vi "生成校准信息.vi"(5 "量程选择":enum16{"低量程", "高量程"}(ring), 7 "公式系数":dbl[](array[numeric]), 8 "启用":bool[](array[boolean]), 9 "校准时间":string[](array[string]), 10 "信号值":dbl[](array[numeric]), 11 "校准浓度":dbl[](array[numeric])) -> ()   [LabVIEW 2016, in "斯坦道CODMn.lvlib"]
panel:
  out "data":T1
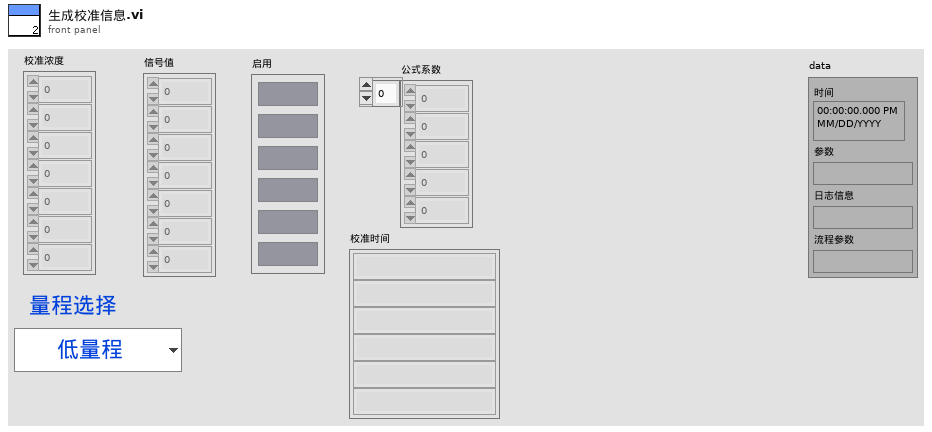
[diagram p1: front panel]
types:
  T1 = typedef "操作日志字段定义.ctl" = cluster{"时间":timestamp, "参数":string, "日志信息":string, "流程参数":string}
  T2 = cluster{"低标液1浓度":dbl, "低标液1信号值":dbl, "低标液1启用":u16, "低标液2浓度":dbl, "低标液2信号值":dbl, "低标液2启用":u16, "低标液3浓度":dbl, "低标液3信号值":dbl, "低标液3启用":u16, "低标液4浓度":dbl, "低标液4信号值":dbl, "低标液4启用":u16, "低标液5浓度":dbl, "低标液5信号值":dbl, "低标液5启用":u16, "高标液1浓度":dbl, "高标液1信号值":dbl, "高标液1启用":u16, "高标液2浓度":dbl, "高标液2信号值":dbl, "高标液2启用":u16, "高标液3浓度":dbl, "高标液3信号值":dbl, "高标液3启用":u16, "高标液4浓度":dbl, "高标液4信号值":dbl, "高标液4启用":u16, "高标液5浓度":dbl, "高标液5信号值":dbl, "高标液5启用":u16}
  T3 = cluster{"[0]":string, "[1]":string, "[2]":string}
  T4 = cluster{"时间标识":timestamp, "参数":string, "日志信息":string, "流程参数":string}
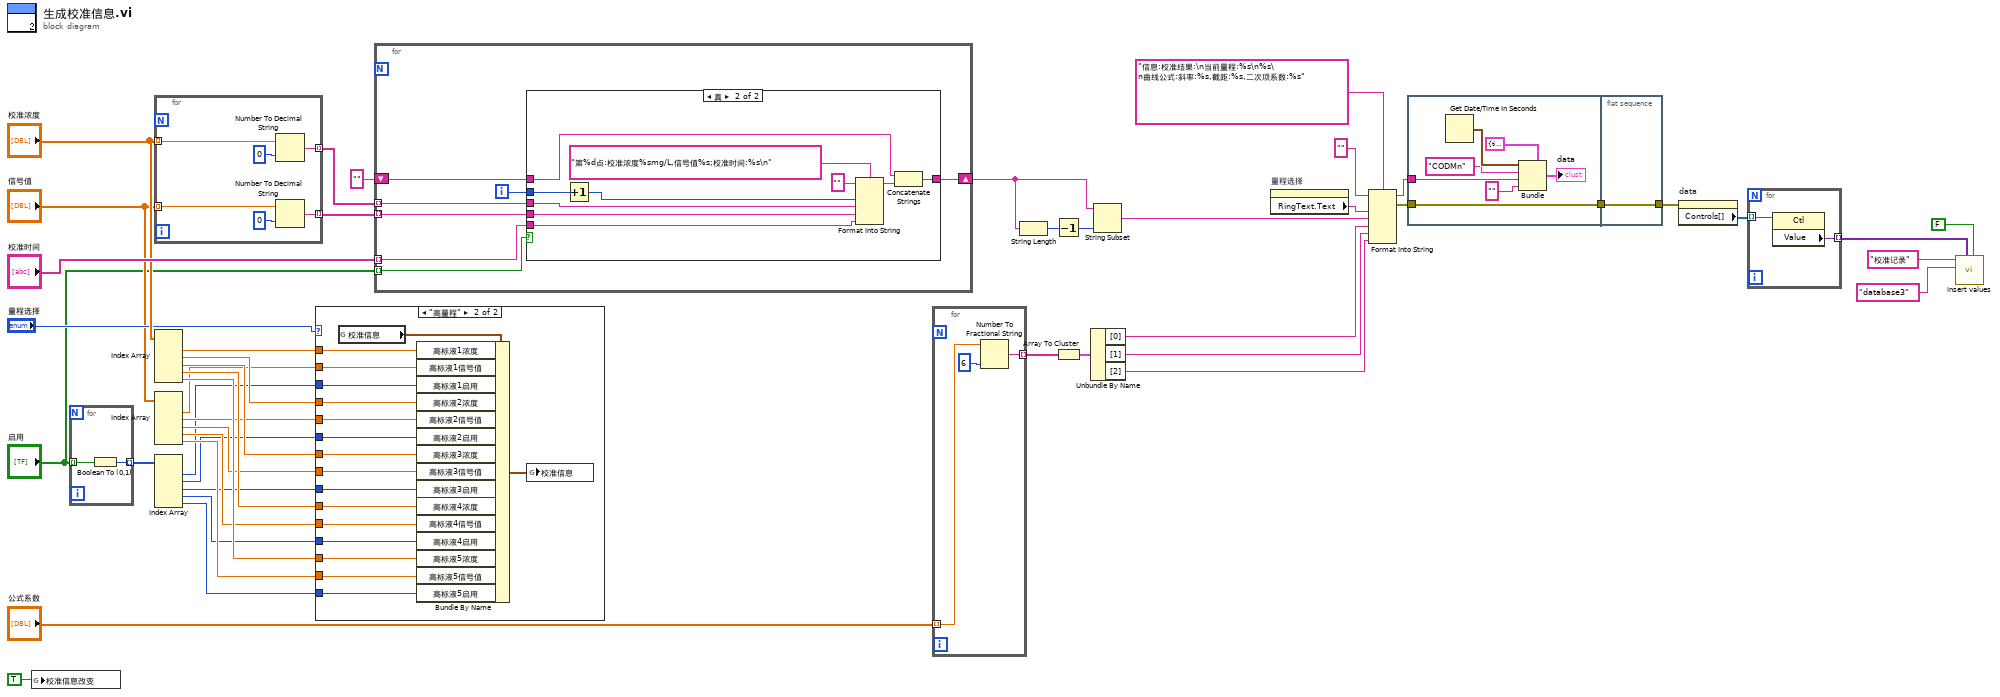
[diagram p0: block diagram]
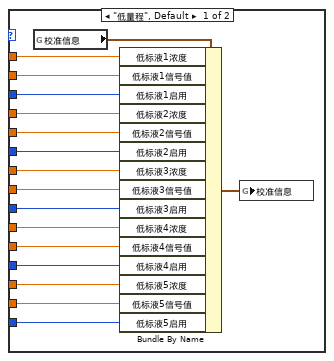
[diagram p2: hidden frame]
diagram:
  n1 = global write "CODMn断电保存全局变量.vi" "校准信息改变"(TRUE ("校准信息改变")) -> ()
  n2 = for {
    tunnel: "启用" -> [w49] mode=indexing
    tunnel: [w48] -> w6 mode=indexing
    n3 = Boolean To (0,1)(Boolean=w49) -> (0, 1=w48:i16)
  }
  n4 = for {
    tunnel: "校准浓度" -> [w55] mode=indexing
    tunnel: "信号值" -> [w52] mode=indexing
    tunnel: [w51] -> w25 mode=indexing
    tunnel: [w50] -> w24 mode=indexing
    n5 = Number To Decimal String(number=w55, width (-)=i16 0 ("宽度(-)")) -> (decimal integer string=w51:string)
    n6 = Number To Decimal String(number=w52, width (-)=i16 0 ("宽度(-)")) -> (decimal integer string=w50:string)
  }
  n7 = Index Array(array="校准浓度") -> (element #1=w18:dbl, element #2=w17:dbl, element #3=w16:dbl, element #4=w15:dbl, element #5=w14:dbl)  [unwired: 5 in]
  n8 = Index Array(array="信号值") -> (element #1=w12:dbl, element #2=w11:dbl, element #3=w10:dbl, element #4=w9:dbl, element #5=w8:dbl)  [unwired: 5 in]
  n9 = Index Array(array=w6) -> (element #1=w5:i16, element #2=w4:i16, element #3=w3:i16, element #4=w2:i16, element #5=w1:i16)  [unwired: 5 in]
  n10 = case shown="\"高量程\"" "量程选择" {
    tunnel: w18 -> [w70 w87]
    tunnel: w17 -> [w69 w86]
    tunnel: w16 -> [w68 w85]
    tunnel: w15 -> [w67 w84]
    tunnel: w14 -> [w66 w83]
    tunnel: w12 -> [w65 w78]
    tunnel: w11 -> [w64 w79]
    tunnel: w10 -> [w63 w80]
    tunnel: w9 -> [w62 w81]
    tunnel: w8 -> [w61 w82]
    tunnel: w5 -> [w56 w77]
    tunnel: w4 -> [w57 w76]
    tunnel: w3 -> [w58 w75]
    tunnel: w2 -> [w59 w74]
    tunnel: w1 -> [w60 w73]
    frame "低量程", Default {
      n11 = global read "CODMn断电保存全局变量.vi" "校准信息"() -> (w71:T2)
      n12 = Bundle By Name(cluster=w71, "低标液1浓度"=w70, "低标液1信号值"=w65, "低标液1启用"=w56, "低标液2浓度"=w69, "低标液2信号值"=w64, "低标液2启用"=w57, "低标液3浓度"=w68, "低标液3信号值"=w63, "低标液3启用"=w58, "低标液4浓度"=w67, "低标液4信号值"=w62, "低标液4启用"=w59, "低标液5浓度"=w66, "低标液5信号值"=w61, "低标液5启用"=w60) -> (w72:T2)
      n13 = global write "CODMn断电保存全局变量.vi" "校准信息"(w72) -> ()
    }
    frame "高量程" {
      n14 = global read "CODMn断电保存全局变量.vi" "校准信息"() -> (w88:T2)
      n15 = Bundle By Name(cluster=w88, "高标液1浓度"=w87, "高标液1信号值"=w78, "高标液1启用"=w77, "高标液2浓度"=w86, "高标液2信号值"=w79, "高标液2启用"=w76, "高标液3浓度"=w85, "高标液3信号值"=w80, "高标液3启用"=w75, "高标液4浓度"=w84, "高标液4信号值"=w81, "高标液4启用"=w74, "高标液5浓度"=w83, "高标液5信号值"=w82, "高标液5启用"=w73) -> (w89:T2)
      n16 = global write "CODMn断电保存全局变量.vi" "校准信息"(w89) -> ()
    }
  }
  n17 = for {
    tunnel: "启用" -> [w96] mode=indexing
    tunnel: w25 -> [w94] mode=indexing
    tunnel: w24 -> [w93] mode=indexing
    shift-right: [w92] -> w44
    shift-left: "" -> [w91]
    tunnel: "校准时间" -> [w90] mode=indexing
    i -> [w95]
    n18 = case shown="真" w96 {
      tunnel: w95 -> [_ w105]
      tunnel: w94 -> [_ w104]
      tunnel: w93 -> [_ w103]
      tunnel: [w97 w100] -> w92
      tunnel: w91 -> [w97 w99]
      tunnel: w90 -> [_ w98]
      frame False {
      }
      frame True {
        n19 = Increment(x=w105) -> (x+1=w106:i32)
        n20 = Format Into String(format string="第%d点:校准浓度%smg/L,信号值%s;校准时间:%s\n" ("格式字符串"), initial string="" ("初始字符串"), w106, w104, w103, w98) -> (resulting string=w101:string)  [unwired: 1 in, 1 out]
        n21 = Concatenate Strings(w99, w101) -> (w100:string)
      }
    }
  }
  n22 = for {
    tunnel: "公式系数" -> [w110] mode=indexing
    tunnel: [w109] -> w23 mode=indexing
    n23 = Number To Fractional String(number=w110, precision (6)=i16 6 ("宽度(-)")) -> (F-format string=w109:string)  [unwired: 2 in]
  }
  n24 = String Length(string=w44) -> (length=w43:i32)
  n25 = Decrement(x=w43) -> (x-1=w42:i32)
  n26 = Array To Cluster(array=w23) -> (cluster=w21:T3)
  n27 = Unbundle By Name(w21) -> ("[0]"=w40:string, "[1]"=w39:string, "[2]"=w38:string)
  n28 = String Subset(string=w44, length (rest)=w42) -> (substring=w37:string)  [unwired: 1 in]
  n29 = property on="量程选择" class="Enum (严格)"() -> ("RingText.Text"=w36:string)  [unwired: 2 in, 2 out]
  n30 = Format Into String(format string="信息:校准结果:\n当前量程:%s\n%s\n曲线公式:斜率:%s,截距:%s,二次项系数:%s", initial string="" ("初始字符串"), w36, w37, w40, w39, w38) -> (resulting string=w30:string, error out=w28:errorcluster)  [unwired: 1 in]
  n31 = flat-sequence {
    tunnel: w30 -> [w113]
    tunnel: [w111] -> w29
    tunnel: w28 -> [w111]
    tunnel: w29 -> [w118]
    tunnel: [w118] -> w27
    frame #0 {
      n32 = Get Date/Time In Seconds() -> (seconds since 1Jan1904=w115:timestamp)
      n33 = Bundle(cluster=T4 {"时间标识"=timestamp(0 s since 1904-01-01), "参数"="", "日志信息"="", "流程参数"=""} ("data in"), "时间标识"=w115, "参数"="CODMn" ("table输入"), "日志信息"=w113, "流程参数"="" ("table输入")) -> (→"data":T4)
    }
    frame #1 {
    }
  }
  n34 = property on="data" class="Clust (严格)"(error in=w27) -> ("Controls[]"=w31:refnum<vi>[])  [unwired: 1 in, 2 out]
  n35 = for {
    tunnel: w31 -> [w120] mode=indexing
    tunnel: [w119] -> w35 mode=indexing
    n36 = property class="Ctl"(reference=w120) -> ("Value"=w119:variant)  [unwired: 1 in, 2 out]
  }
  n37 = call "insert values.vi"("是否创建唯一键"=FALSE, "data"=w35, "database"="database3", "Tabe Name"="校准记录") -> ()  [unwired: 7 in, 1 out]
